vi "CVT Init.vi"(8 "error in (no error)":errorcluster, 11 "Tag List":T1[](array[typedef])) -> (0 "error out":errorcluster)   [LabVIEW 2010]
uses:
  _SubVIs/TypeDefs/cvt_Tag Configuration.ctl
  _SubVIs/TypeDefs/cvt_Data Types.ctl
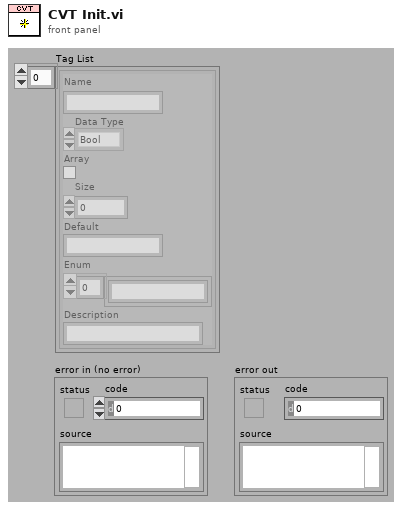
[diagram p1: front panel]
types:
  T1 = typedef "cvt_Tag Configuration.ctl" = cluster{"Name":string, "Data Type":T2, "Array":bool, "Size":u32, "Default":string, "Enum":string[], "Description":string}
  T2 = typedef "cvt_Data Types.ctl" = enum16{"Bool", "U8", "I32", "Double", "String", "Enum"}
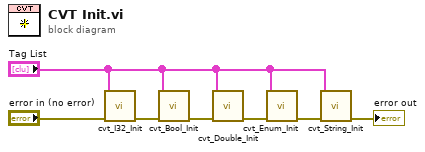
[diagram p0: block diagram]
diagram:
  n1 = call "cvt_I32_Init.vi"("error in (no error)"="error in (no error)", "Tag List"="Tag List") -> ("error out"=w6:errorcluster)  [unwired: 9 out]
  n2 = call "cvt_Bool_Init.vi"("error in (no error)"=w6, "Tag List"="Tag List") -> ("error out"=w7:errorcluster)  [unwired: 9 out]
  n3 = call "cvt_Double_Init.vi"("error in (no error)"=w7, "Tag List"="Tag List") -> ("error out"=w4:errorcluster)  [unwired: 9 out]
  n4 = call "cvt_Enum_Init.vi"("error in (no error)"=w4, "Tag List"="Tag List") -> ("error out"=w2:errorcluster)  [unwired: 9 out]
  n5 = call "cvt_String_Init.vi"("error in (no error)"=w2, "Tag List"="Tag List") -> ("error out"=→"error out":errorcluster)  [unwired: 9 out]
